vi "APS wdt get counter.vi"(8 "error in (no error)":errorcluster caption="错误输入（无错误）", 9 "Counter":i32, 10 "TimerNo":i32, 11 "Board_ID":i32) -> (0 "error out":errorcluster caption="错误输出", 1 "Counter out":i32, 3 "function return":i32)   [LabVIEW 2011, in "APS168.lvlib"]
doc: "I32 FNTYPE APS_wdt_get_counter( I32 Board_ID, I32 TimerNo, I32 *Counter );"
uses:
  APS168.lvlib
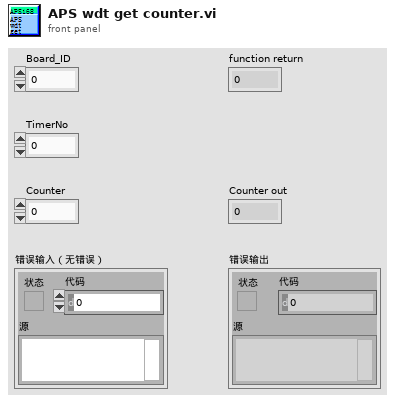
[diagram p1: front panel]
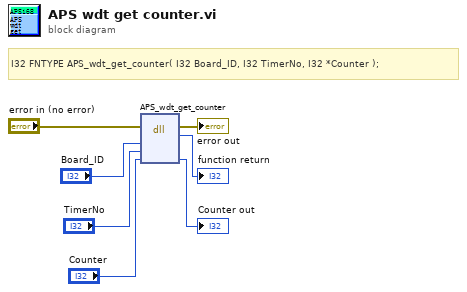
[diagram p0: block diagram]
diagram:
  # "I32 FNTYPE APS_wdt_get_counter( I32 Board_ID, I32 TimerNo, I32 *Counter );"
  n1 = dll-call lib="PTH1Labs E软件ADLINK 204CAPS_1_7_1_LIB line 连续运动204APS168.*" fn="APS_wdt_get_counter"(error in="error in (no error)", "Board_ID"="Board_ID", "TimerNo"="TimerNo", "Counter"="Counter") -> (error out=→"error out":errorcluster, →"function return":i32, "Counter"=→"Counter out":i32)  [unwired: 4 in, 1 out]
